vi "Write Subpanel Events.vi"(8 "error in (no error)":errorcluster, 10 "SubPanel Events":T1, 11 "CIF_UI in":refnum<class "CIF_UI.lvclass">) -> (0 "error out":errorcluster, 3 "CIF_UI out":refnum<class "CIF_UI.lvclass">)   [LabVIEW 2021, in "CIF_UI.lvclass"]
uses:
  CIF_UI.lvclass
  Typedef/SubPanel Events.ctl
  Typedef/New Connection Event Data.ctl
  <vilib>/gRPC/LabVIEW gRPC Library/Shared/grpcId.ctl
  Typedef/New Connection Plugin Event Data.ctl
  CIF_UI.lvclass/CIF_UI.ctl
  <vilib>/gRPC/LabVIEW gRPC Library/grpc-lvsupport-release.lvlib
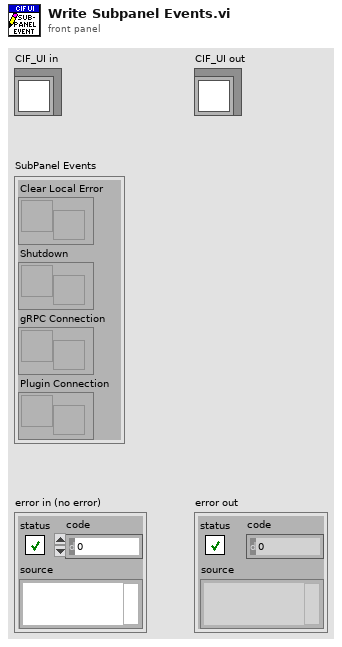
[diagram p1: front panel]
types:
  T1 = typedef "CIF_UI.lvclass/SubPanel Events.ctl" = cluster{"Clear Local Error":refnum<user-event>, "Shutdown":refnum<user-event>, "gRPC Connection":refnum<user-event>, "Plugin Connection":refnum<user-event>}
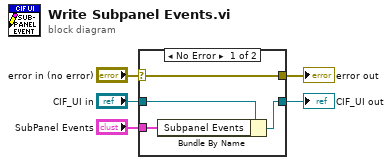
[diagram p0: block diagram]
diagram:
  n1 = case shown="No Error" "error in (no error)" {
    selector: "error in (no error)" -> [w9 w10]
    tunnel: [w9 w10] -> w4
    tunnel: [w7 w11] -> w2
    tunnel: "CIF_UI in" -> [w8 w11]
    tunnel: "SubPanel Events" -> [w6 _]
    frame No Error {
      n2 = Bundle By Name(cluster=w8, "Subpanel Events"=w6) -> (w7:refnum<class "CIF_UI.lvclass">)
    }
    frame Error {
    }
  }
  "error out" <- w4
  "CIF_UI out" <- w2
